vi "SW_Calc_speed.vi"(2 "Y coord, mm":dbl, 3 "X coord, mm":dbl, 4 "Time per frame, s":dbl) -> (0 "Mouse speed, mm/s":dbl, 1 "Mouse speed, mm/s":string)   [LabVIEW 2016]
doc: "This VI calculates speed using smoothing of the input noisy data according to Holoborodko' algorithm: http://www.holoborodko.com/pavel/numerical-methods/numerical-derivative/smooth-low-noise-differentiator"
panel:
  in  "Speed smoothing type":u16(ring)=3 items=["None", "Holoborodko 2/5", "Holoborodko 2/7", "Holoborodko 2/11", "Holoborodko 4/7"]
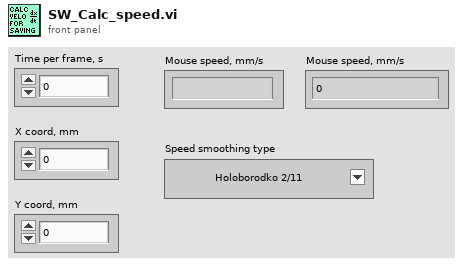
[diagram p1: front panel]
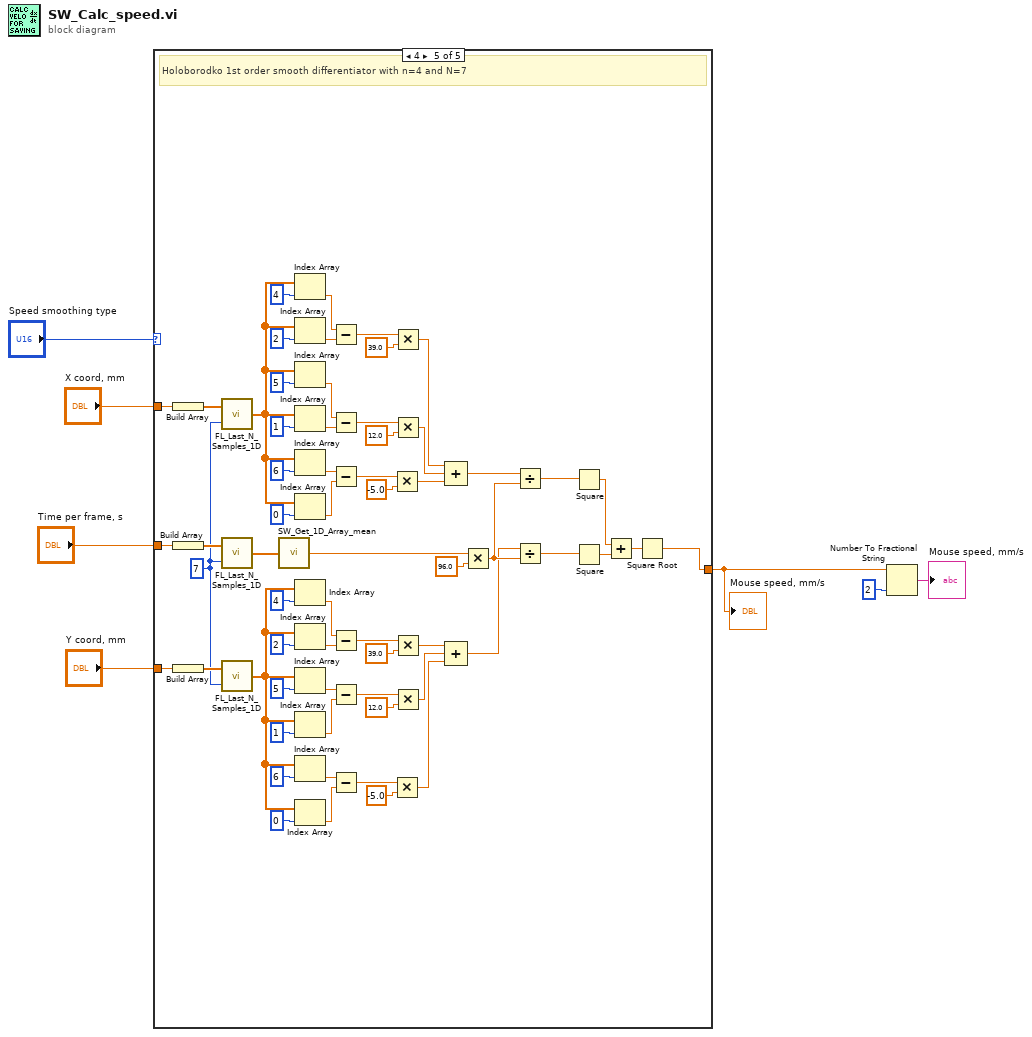
[diagram p0: block diagram]
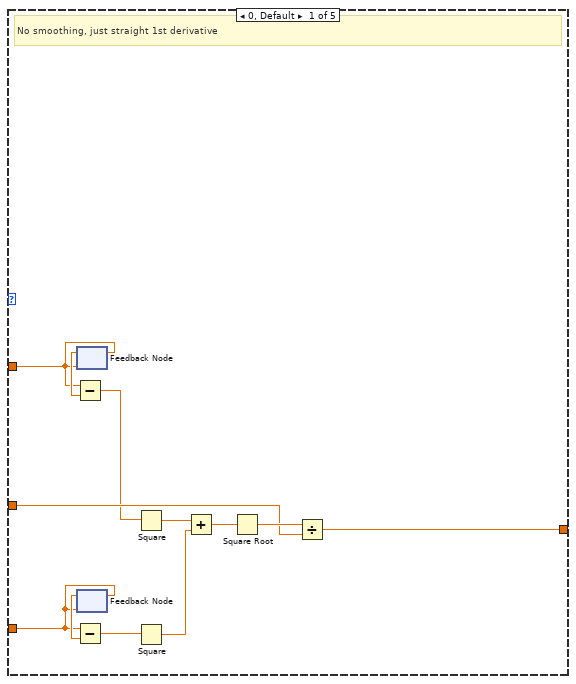
[diagram p2: hidden frame]
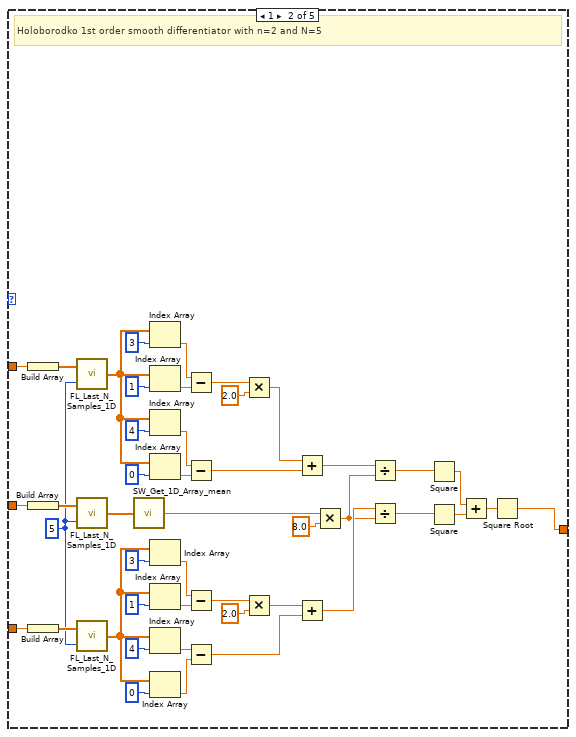
[diagram p3: hidden frame]
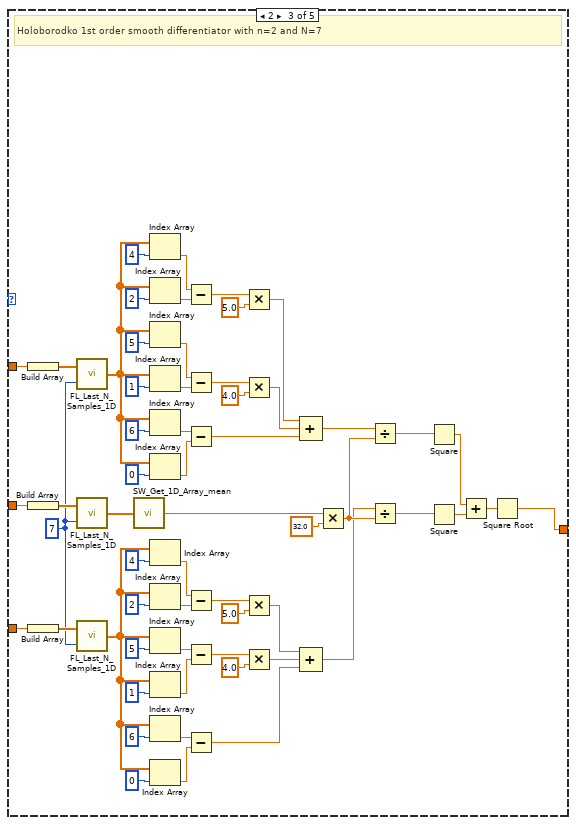
[diagram p4: hidden frame]
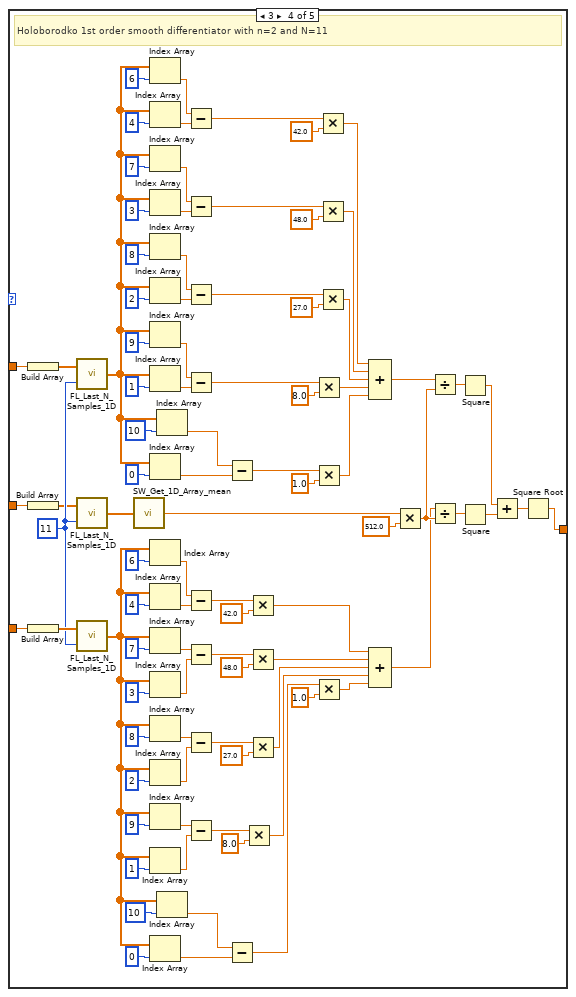
[diagram p5: hidden frame]
diagram:
  n1 = case shown="4" "Speed smoothing type" {
    tunnel: "Time per frame, s" -> [w15 w64 w123 w127 w277]
    tunnel: "Y coord, mm" -> [w9 w60 w119 w212 w273]
    tunnel: "X coord, mm" -> [w11 w59 w118 w211 w272]
    tunnel: [w14 w22 w101 w194 w255] -> w6
    frame 0, Default {
      # "No smoothing, just straight 1st derivative"
      n2 = feedback #1(w11) -> (w12:dbl)
      n3 = Subtract(x=w11, y=w12) -> (x-y=w10:dbl)
      n4 = feedback-in #1(w11) -> ()
      n5 = feedback #2(w9) -> (w13:dbl)
      n6 = Subtract(x=w9, y=w13) -> (x-y=w8:dbl)
      n7 = feedback-in #2(w9) -> ()
      n8 = Square(x=w10) -> (x^2=w18:dbl)
      n9 = Square(x=w8) -> (x^2=w19:dbl)
      n10 = Add(x=w18, y=w19) -> (x+y=w17:dbl)
      n11 = Square Root(x=w17) -> (sqrt(x)=w16:dbl)
      n12 = Divide(x=w16, y=w15) -> (x/y=w14:dbl)
    }
    frame 1 {
      w58 = u32 5 ("BufferLengthSamples")
      # "Holoborodko 1st order smooth differentiator with n=2 and N=5"
      n13 = Build Array(w59) -> (w62:dbl[])
      n14 = Build Array(w64) -> (w63:dbl[])
      n15 = Build Array(w60) -> (w61:dbl[])
      n16 = call "FL_Last_N_Samples_1D.vi"("BufferLengthSamples"=w58, "Input Array of strings"=w62) -> ("Output Array of strings"=w49:dbl[])
      n17 = call "FL_Last_N_Samples_1D.vi"("BufferLengthSamples"=w58, "Input Array of strings"=w63) -> ("Output Array of strings"=w21:dbl[])
      n18 = call "FL_Last_N_Samples_1D.vi"("BufferLengthSamples"=w58, "Input Array of strings"=w61) -> ("Output Array of strings"=w29:dbl[])
      n19 = call "SW_Get_1D_Array_mean.vi"("1D array"=w21) -> ("Mean of 1D Array"=w20:dbl)
      n20 = Index Array(array=w49, index=3) -> (element=w55:dbl)
      n21 = Index Array(array=w49, index=1) -> (element=w54:dbl)
      n22 = Index Array(array=w49, index=4) -> (element=w48:dbl)
      n23 = Index Array(array=w49, index=0) -> (element=w47:dbl)
      n24 = Index Array(array=w29, index=3) -> (element=w32:dbl)
      n25 = Index Array(array=w29, index=1) -> (element=w33:dbl)
      n26 = Index Array(array=w29, index=4) -> (element=w38:dbl)
      n27 = Index Array(array=w29, index=0) -> (element=w39:dbl)
      n28 = Subtract(x=w55, y=w54) -> (x-y=w53:dbl)
      n29 = Subtract(x=w48, y=w47) -> (x-y=w45:dbl)
      n30 = Subtract(x=w32, y=w33) -> (x-y=w34:dbl)
      n31 = Subtract(x=w38, y=w39) -> (x-y=w41:dbl)
      n32 = Multiply(x=w53, y=2.0) -> (x*y=w46:dbl)
      n33 = Multiply(x=w34, y=2.0) -> (x*y=w40:dbl)
      n34 = Add(x=w46, y=w45) -> (x+y=w44:dbl)
      n35 = Add(x=w40, y=w41) -> (x+y=w42:dbl)
      n36 = Multiply(x=w20, y=8.0) -> (x*y=w28:dbl)
      n37 = Divide(x=w44, y=w28) -> (x/y=w25:dbl)
      n38 = Divide(x=w42, y=w28) -> (x/y=w23:dbl)
      n39 = Square(x=w25) -> (x^2=w24:dbl)
      n40 = Square(x=w23) -> (x^2=w26:dbl)
      n41 = Add(x=w24, y=w26) -> (x+y=w27:dbl)
      n42 = Square Root(x=w27) -> (sqrt(x)=w22:dbl)
    }
    frame 2 {
      w117 = u32 7 ("BufferLengthSamples")
      # "Holoborodko 1st order smooth differentiator with n=2 and N=7"
      n43 = Build Array(w118) -> (w121:dbl[])
      n44 = Build Array(w123) -> (w122:dbl[])
      n45 = Build Array(w119) -> (w120:dbl[])
      n46 = call "FL_Last_N_Samples_1D.vi"("BufferLengthSamples"=w117, "Input Array of strings"=w121) -> ("Output Array of strings"=w96:dbl[])
      n47 = call "FL_Last_N_Samples_1D.vi"("BufferLengthSamples"=w117, "Input Array of strings"=w122) -> ("Output Array of strings"=w66:dbl[])
      n48 = call "FL_Last_N_Samples_1D.vi"("BufferLengthSamples"=w117, "Input Array of strings"=w120) -> ("Output Array of strings"=w69:dbl[])
      n49 = call "SW_Get_1D_Array_mean.vi"("1D array"=w66) -> ("Mean of 1D Array"=w65:dbl)
      n50 = Index Array(array=w96, index=4) -> (element=w114:dbl)
      n51 = Index Array(array=w96, index=2) -> (element=w113:dbl)
      n52 = Index Array(array=w96, index=5) -> (element=w110:dbl)
      n53 = Index Array(array=w96, index=1) -> (element=w109:dbl)
      n54 = Index Array(array=w96, index=6) -> (element=w99:dbl)
      n55 = Index Array(array=w96, index=0) -> (element=w100:dbl)
      n56 = Index Array(array=w69, index=4) -> (element=w72:dbl)
      n57 = Index Array(array=w69, index=2) -> (element=w73:dbl)
      n58 = Index Array(array=w69, index=5) -> (element=w76:dbl)
      n59 = Index Array(array=w69, index=1) -> (element=w77:dbl)
      n60 = Index Array(array=w69, index=6) -> (element=w79:dbl)
      n61 = Index Array(array=w69, index=0) -> (element=w78:dbl)
      n62 = Subtract(x=w114, y=w113) -> (x-y=w95:dbl)
      n63 = Subtract(x=w110, y=w109) -> (x-y=w93:dbl)
      n64 = Subtract(x=w99, y=w100) -> (x-y=w91:dbl)
      n65 = Subtract(x=w72, y=w73) -> (x-y=w82:dbl)
      n66 = Subtract(x=w76, y=w77) -> (x-y=w84:dbl)
      n67 = Subtract(x=w79, y=w78) -> (x-y=w86:dbl)
      n68 = Multiply(x=w95, y=5.0) -> (x*y=w89:dbl)
      n69 = Multiply(x=w93, y=4.0) -> (x*y=w90:dbl)
      n70 = Multiply(x=w82, y=5.0) -> (x*y=w88:dbl)
      n71 = Multiply(x=w84, y=4.0) -> (x*y=w87:dbl)
      n72 = Compound Arithmetic op=ADD(w89, w90, w91) -> (w68:dbl)
      n73 = Compound Arithmetic op=ADD(w88, w87, w86) -> (w67:dbl)
      n74 = Multiply(x=w65, y=32.0) -> (x*y=w107:dbl)
      n75 = Divide(x=w68, y=w107) -> (x/y=w104:dbl)
      n76 = Divide(x=w67, y=w107) -> (x/y=w102:dbl)
      n77 = Square(x=w104) -> (x^2=w103:dbl)
      n78 = Square(x=w102) -> (x^2=w105:dbl)
      n79 = Add(x=w103, y=w105) -> (x+y=w106:dbl)
      n80 = Square Root(x=w106) -> (sqrt(x)=w101:dbl)
    }
    frame 3 {
      w210 = u32 11 ("BufferLengthSamples")
      # "Holoborodko 1st order smooth differentiator with n=2 and N=11"
      n81 = Build Array(w211) -> (w214:dbl[])
      n82 = Build Array(w127) -> (w126:dbl[])
      n83 = Build Array(w212) -> (w213:dbl[])
      n84 = call "FL_Last_N_Samples_1D.vi"("BufferLengthSamples"=w210, "Input Array of strings"=w214) -> ("Output Array of strings"=w167:dbl[])
      n85 = call "FL_Last_N_Samples_1D.vi"("BufferLengthSamples"=w210, "Input Array of strings"=w126) -> ("Output Array of strings"=w125:dbl[])
      n86 = call "FL_Last_N_Samples_1D.vi"("BufferLengthSamples"=w210, "Input Array of strings"=w213) -> ("Output Array of strings"=w129:dbl[])
      n87 = call "SW_Get_1D_Array_mean.vi"("1D array"=w125) -> ("Mean of 1D Array"=w124:dbl)
      n88 = Index Array(array=w167, index=6) -> (element=w207:dbl)
      n89 = Index Array(array=w167, index=4) -> (element=w206:dbl)
      n90 = Index Array(array=w167, index=7) -> (element=w203:dbl)
      n91 = Index Array(array=w167, index=3) -> (element=w202:dbl)
      n92 = Index Array(array=w167, index=8) -> (element=w192:dbl)
      n93 = Index Array(array=w167, index=2) -> (element=w193:dbl)
      n94 = Index Array(array=w167, index=9) -> (element=w175:dbl)
      n95 = Index Array(array=w167, index=1) -> (element=w174:dbl)
      n96 = Index Array(array=w167, index=0) -> (element=w173:dbl)
      n97 = Index Array(array=w129, index=6) -> (element=w132:dbl)
      n98 = Index Array(array=w129, index=4) -> (element=w133:dbl)
      n99 = Index Array(array=w129, index=7) -> (element=w136:dbl)
      n100 = Index Array(array=w129, index=3) -> (element=w137:dbl)
      n101 = Index Array(array=w129, index=8) -> (element=w139:dbl)
      n102 = Index Array(array=w129, index=2) -> (element=w138:dbl)
      n103 = Index Array(array=w129, index=9) -> (element=w155:dbl)
      n104 = Index Array(array=w129, index=1) -> (element=w156:dbl)
      n105 = Index Array(array=w129, index=0) -> (element=w157:dbl)
      n106 = Index Array(array=w167, index=10) -> (element=w172:dbl)
      n107 = Index Array(array=w129, index=10) -> (element=w158:dbl)
      n108 = Subtract(x=w207, y=w206) -> (x-y=w189:dbl)
      n109 = Subtract(x=w203, y=w202) -> (x-y=w187:dbl)
      n110 = Subtract(x=w192, y=w193) -> (x-y=w185:dbl)
      n111 = Subtract(x=w175, y=w174) -> (x-y=w178:dbl)
      n112 = Subtract(x=w132, y=w133) -> (x-y=w142:dbl)
      n113 = Subtract(x=w136, y=w137) -> (x-y=w144:dbl)
      n114 = Subtract(x=w139, y=w138) -> (x-y=w146:dbl)
      n115 = Subtract(x=w155, y=w156) -> (x-y=w152:dbl)
      n116 = Subtract(x=w172, y=w173) -> (x-y=w169:dbl)
      n117 = Subtract(x=w158, y=w157) -> (x-y=w161:dbl)
      n118 = Multiply(x=w152, y=8.0) -> (x*y=w163:dbl)
      n119 = Multiply(x=w142, y=42.0) -> (x*y=w148:dbl)
      n120 = Multiply(x=w144, y=48.0) -> (x*y=w147:dbl)
      n121 = Multiply(x=w146, y=27.0) -> (x*y=w149:dbl)
      n122 = Multiply(x=w178, y=8.0) -> (x*y=w166:dbl)
      n123 = Multiply(x=w169, y=1.0) -> (x*y=w165:dbl)
      n124 = Multiply(x=w161, y=1.0) -> (x*y=w164:dbl)
      n125 = Multiply(x=w189, y=42.0) -> (x*y=w183:dbl)
      n126 = Multiply(x=w187, y=48.0) -> (x*y=w184:dbl)
      n127 = Multiply(x=w185, y=27.0) -> (x*y=w181:dbl)
      n128 = Compound Arithmetic op=ADD(w183, w184, w181, w166, w165) -> (w182:dbl)
      n129 = Compound Arithmetic op=ADD(w148, w147, w149, w163, w164) -> (w128:dbl)
      n130 = Multiply(x=w124, y=512.0) -> (x*y=w200:dbl)
      n131 = Divide(x=w182, y=w200) -> (x/y=w197:dbl)
      n132 = Divide(x=w128, y=w200) -> (x/y=w195:dbl)
      n133 = Square(x=w197) -> (x^2=w196:dbl)
      n134 = Square(x=w195) -> (x^2=w198:dbl)
      n135 = Add(x=w196, y=w198) -> (x+y=w199:dbl)
      n136 = Square Root(x=w199) -> (sqrt(x)=w194:dbl)
    }
    frame 4 {
      w271 = u32 7 ("BufferLengthSamples")
      # "Holoborodko 1st order smooth differentiator with n=4 and N=7"
      n137 = Build Array(w272) -> (w275:dbl[])
      n138 = Build Array(w277) -> (w276:dbl[])
      n139 = Build Array(w273) -> (w274:dbl[])
      n140 = call "FL_Last_N_Samples_1D.vi"("BufferLengthSamples"=w271, "Input Array of strings"=w275) -> ("Output Array of strings"=w250:dbl[])
      n141 = call "FL_Last_N_Samples_1D.vi"("BufferLengthSamples"=w271, "Input Array of strings"=w276) -> ("Output Array of strings"=w216:dbl[])
      n142 = call "FL_Last_N_Samples_1D.vi"("BufferLengthSamples"=w271, "Input Array of strings"=w274) -> ("Output Array of strings"=w223:dbl[])
      n143 = call "SW_Get_1D_Array_mean.vi"("1D array"=w216) -> ("Mean of 1D Array"=w215:dbl)
      n144 = Index Array(array=w250, index=4) -> (element=w268:dbl)
      n145 = Index Array(array=w250, index=2) -> (element=w267:dbl)
      n146 = Index Array(array=w250, index=5) -> (element=w264:dbl)
      n147 = Index Array(array=w250, index=1) -> (element=w263:dbl)
      n148 = Index Array(array=w250, index=6) -> (element=w253:dbl)
      n149 = Index Array(array=w250, index=0) -> (element=w254:dbl)
      n150 = Index Array(array=w223, index=4) -> (element=w226:dbl)
      n151 = Index Array(array=w223, index=2) -> (element=w227:dbl)
      n152 = Index Array(array=w223, index=5) -> (element=w230:dbl)
      n153 = Index Array(array=w223, index=1) -> (element=w231:dbl)
      n154 = Index Array(array=w223, index=6) -> (element=w233:dbl)
      n155 = Index Array(array=w223, index=0) -> (element=w232:dbl)
      n156 = Subtract(x=w268, y=w267) -> (x-y=w249:dbl)
      n157 = Subtract(x=w264, y=w263) -> (x-y=w247:dbl)
      n158 = Subtract(x=w253, y=w254) -> (x-y=w245:dbl)
      n159 = Subtract(x=w226, y=w227) -> (x-y=w236:dbl)
      n160 = Subtract(x=w230, y=w231) -> (x-y=w238:dbl)
      n161 = Subtract(x=w233, y=w232) -> (x-y=w240:dbl)
      n162 = Multiply(x=w245, y=-5.0) -> (x*y=w220:dbl)
      n163 = Multiply(x=w240, y=-5.0) -> (x*y=w218:dbl)
      n164 = Multiply(x=w249, y=39.0) -> (x*y=w243:dbl)
      n165 = Multiply(x=w247, y=12.0) -> (x*y=w244:dbl)
      n166 = Multiply(x=w236, y=39.0) -> (x*y=w242:dbl)
      n167 = Multiply(x=w238, y=12.0) -> (x*y=w241:dbl)
      n168 = Compound Arithmetic op=ADD(w243, w244, w220) -> (w222:dbl)
      n169 = Compound Arithmetic op=ADD(w242, w241, w218) -> (w221:dbl)
      n170 = Multiply(x=w215, y=96.0) -> (x*y=w261:dbl)
      n171 = Divide(x=w222, y=w261) -> (x/y=w258:dbl)
      n172 = Divide(x=w221, y=w261) -> (x/y=w256:dbl)
      n173 = Square(x=w258) -> (x^2=w257:dbl)
      n174 = Square(x=w256) -> (x^2=w259:dbl)
      n175 = Add(x=w257, y=w259) -> (x+y=w260:dbl)
      n176 = Square Root(x=w260) -> (sqrt(x)=w255:dbl)
    }
  }
  "Mouse speed, mm/s" <- w6
  n177 = Number To Fractional String(number=w6, precision (6)=i16 2) -> (F-format string=→"Mouse speed, mm/s":string)  [unwired: 2 in]
